vi "Voltage and Current Ring Chooser.vi"(8 "error in (no error)":errorcluster, 11 "Yokogawa WT2X0 in":refnum<class "Yokogawa WT2X0.lvclass">) -> (0 "error out":errorcluster, 1 "Current Strings And Values []":T1, 2 "Voltage Strings And Values []":T1, 3 "Yokogawa WT2X0 out":refnum<class "Yokogawa WT2X0.lvclass">, 4 "Wiring Strings And Values []":T1)   [LabVIEW 2013, in "Universal Power Meter.lvlib" / "Yokogawa WT2X0.lvlib" / "Yokogawa WT2X0.lvclass"]
uses:
  Yokogawa WT2X0.lvclass
  <vilib>/Utility/miscctls.llb/LVStringsAndValuesArrayTypeDef_U16.ctl
panel:
  in  "Wiring (1: 1P3W)":u16(ring)=1 items=["1P3W", "3P3W", "3P4W", "3V3A"]
  in  "A Range (12: 20A)":u16(ring)=12 items=["Auto", "5mA", "10mA", "20mA", "50mA", "100mA", "200mA", "0.5A", "1A", "2A", "5A", "10A", "20A", "50mV", "100mV", "200mV", "2.5V", "5V", "10V"]
  in  "V Range (6: 600V)":u16(ring)=6 items=["Auto", "15V", "30V", "60V", "150V", "300V", "600V"]
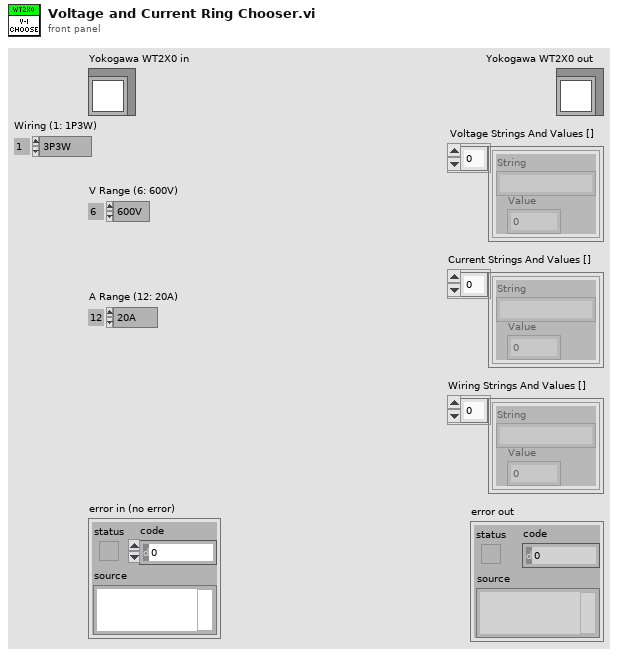
[diagram p1: front panel]
types:
  T1 = typedef "LVStringsAndValuesArrayTypeDef_U16.ctl" = cluster{"String":string, "Value":u16}[]
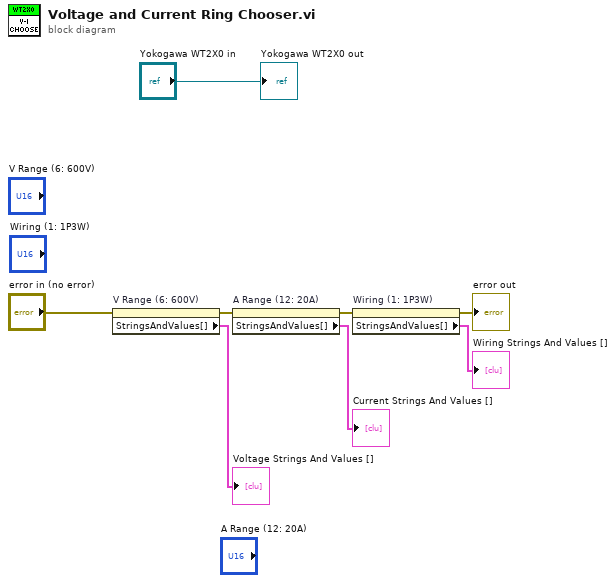
[diagram p0: block diagram]
diagram:
  n1 = property on="V Range (6: 600V)" class="Ring (strict)"(error in="error in (no error)") -> (error out=w4:errorcluster, "StringsAndValues[]"=→"Voltage Strings And Values []":T1)  [unwired: 1 in, 1 out]
  n2 = property on="A Range (12: 20A)" class="Ring (strict)"(error in=w4) -> (error out=w3:errorcluster, "StringsAndValues[]"=→"Current Strings And Values []":T1)  [unwired: 1 in, 1 out]
  n3 = property on="Wiring (1: 1P3W)" class="Ring (strict)"(error in=w3) -> (error out=→"error out":errorcluster, "StringsAndValues[]"=→"Wiring Strings And Values []":T1)  [unwired: 1 in, 1 out]
  "Yokogawa WT2X0 out" <- "Yokogawa WT2X0 in"
